vi "控制.vi"(8 "error in (no error)":errorcluster caption="错误输入（无错误）", 11 "信号灯成员类 输入":refnum<class "信号灯成员类.lvclass">) -> (0 "error out":errorcluster caption="错误输出", 3 "信号灯成员类 输出":refnum<class "信号灯成员类.lvclass">)   [LabVIEW 2017, in "信号灯成员类.lvclass"]
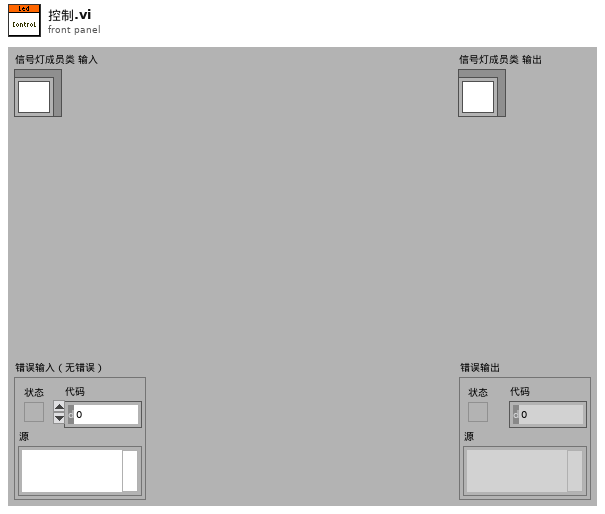
[diagram p1: front panel]
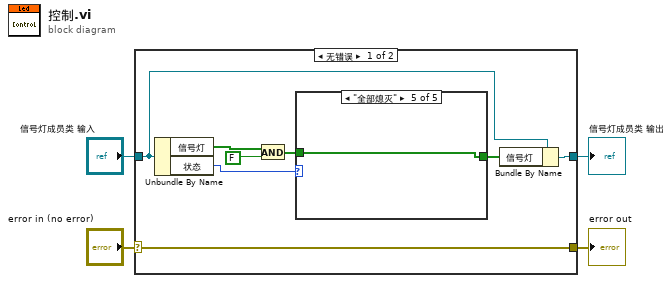
[diagram p0: block diagram]
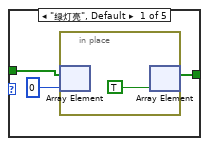
[diagram p2: hidden frame]
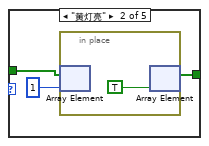
[diagram p3: hidden frame]
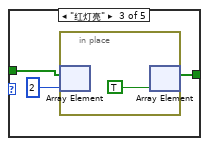
[diagram p4: hidden frame]
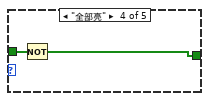
[diagram p5: hidden frame]
diagram:
  n1 = case shown="无错误" "error in (no error)" {
    selector: "error in (no error)" -> [w12 w29]
    tunnel: [w12 w29] -> w3
    tunnel: [w5 w28] -> w1
    tunnel: "信号灯成员类 输入" -> [w6 w28]
    frame No Error {
      n2 = Unbundle By Name(w6) -> ("信号灯"=w9:bool[], "状态"=w11:enum16{"绿灯亮", "黄灯亮", "红灯亮", "全部亮", "全部熄灭"})
      n3 = And(x=w9, y=FALSE) -> (x .and. y?=w8:bool[])
      n4 = case shown="\"全部熄灭\"" w11 {
        tunnel: w8 -> [w14 w19 w21 w26 w27]
        tunnel: [w13 w17 w22 w25 w27] -> w7
        frame "绿灯亮", Default {
          n5 = in-place {
            n6 = in-place-array #1(w14, 0) -> ()  [unwired: 1 out]
            n7 = in-place-array #1(TRUE ("元素")) -> (w13:bool[])  [unwired: 1 out]
          }
        }
        frame "黄灯亮" {
          n8 = in-place {
            n9 = in-place-array #2(w19, 1) -> ()  [unwired: 1 out]
            n10 = in-place-array #2(TRUE ("元素")) -> (w17:bool[])  [unwired: 1 out]
          }
        }
        frame "红灯亮" {
          n11 = in-place {
            n12 = in-place-array #3(w21, 2) -> ()  [unwired: 1 out]
            n13 = in-place-array #3(TRUE ("元素")) -> (w22:bool[])  [unwired: 1 out]
          }
        }
        frame "全部亮" {
          n14 = Not(x=w26) -> (.not. x?=w25:bool[])
        }
        frame "全部熄灭" {
        }
      }
      n15 = Bundle By Name(cluster=w6, "信号灯"=w7) -> (w5:refnum<class "信号灯成员类.lvclass">)
    }
    frame Error {
    }
  }
  "error out" <- w3
  "信号灯成员类 输出" <- w1
